vi "cmdCode2Text.vi"(1 "CommandCode":string) -> (0 "CommandText":T1)   [LabVIEW 2010]
uses:
  OutputDataFormat.ctl
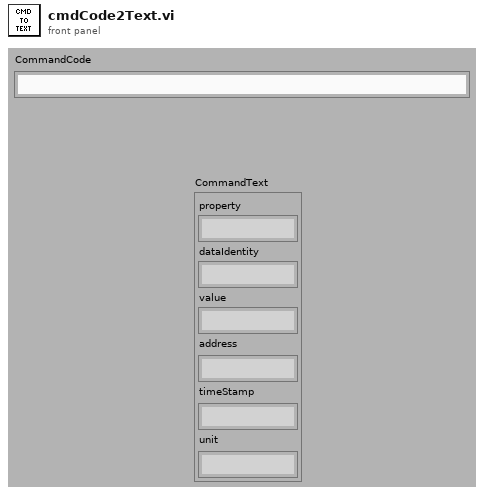
[diagram p1: front panel]
types:
  T1 = typedef "OutputDataFormat.ctl" = cluster{"property":string, "dataIdentity":string, "value":string, "address":string, "timeStamp":string, "unit":string}
  T2 = cluster{"address":string, "controlCode":string, "dataLength":dbl, "dataSection":string, "checkCode":string}
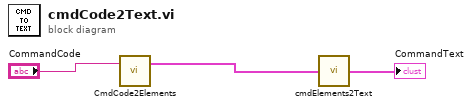
[diagram p0: block diagram]
diagram:
  n1 = call "CmdCode2Elements.vi"("CommandCode"="CommandCode") -> ("Elements"=w3:T2)  [unwired: 1 in, 1 out]
  n2 = call "cmdElements2Text.vi"("CodeElements"=w3) -> ("CommandText"=→"CommandText":T1)
